vi "DI Read Body.vi"(6 "error in":errorcluster, 9 "Channel":tag) -> (0 "error out":errorcluster, 2 "data":bool)   [LabVIEW 2015, in "DAQ.lvlib"]
uses:
  DAQ.lvlib
  <vilib>/DAQmx/read.llb/DAQmx Read (Digital Bool 1Line 1Point).vi
  <vilib>/DAQmx/create/channels.llb/DAQmx Create Channel (DI-Digital Input).vi
  <vilib>/DAQmx/miscellaneous.llb/DAQmx Fill In Error Info.vi
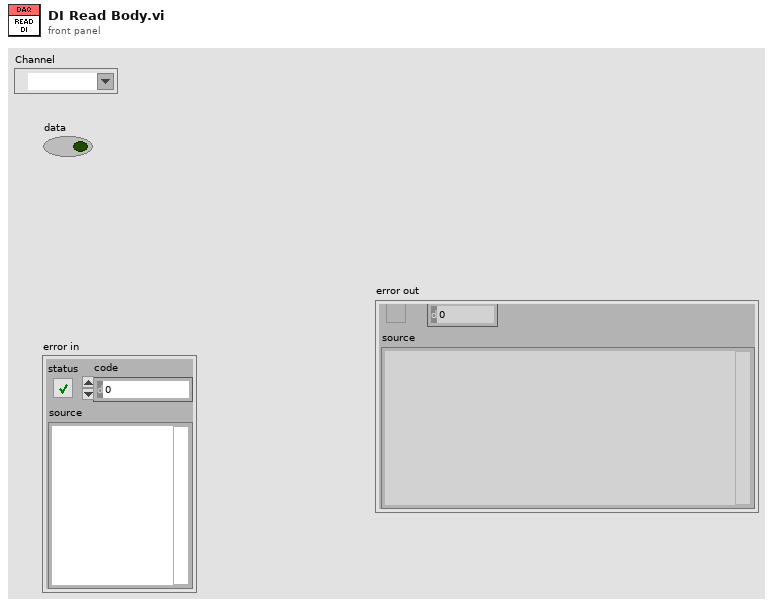
[diagram p1: front panel]
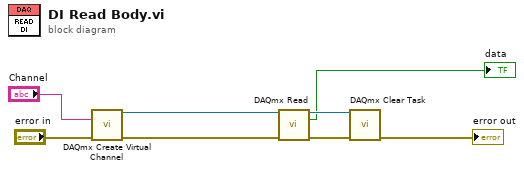
[diagram p0: block diagram]
diagram:
  n1 = call-poly <vilib>:"DAQmx Create Virtual Channel.vi"("lines"="Channel", "error in"="error in") -> ("task out"=w5:refnum<k21>, "error out"=w3:errorcluster)  [unwired: 12 in]
  n2 = call-poly <vilib>:"DAQmx Read.vi"("task/channels in"=w5, "error in"=w3) -> ("task out"=w4:refnum<k21>, "data"=→"data":bool, "error out"=w2:errorcluster)  [unwired: 11 in]
  n3 = call <vilib>:"DAQmx Clear Task.vi"("task in"=w4, "error in"=w2) -> ("error out"=→"error out":errorcluster)  [unwired: 13 in]
